vi "Time Delay.vi"(0 "Waiting Time(S)":u32, 1 "Pop Messige":string="Time Remaining:", 3 "error in (no error)":errorcluster) -> (10 "error out":errorcluster)   [LabVIEW 2020]
panel:
  out "String":string
  out "Horizontal Progress Bar":u32(slide) min=30 max=30000 scale=-1.0..10.0
  in  "Stop":bool
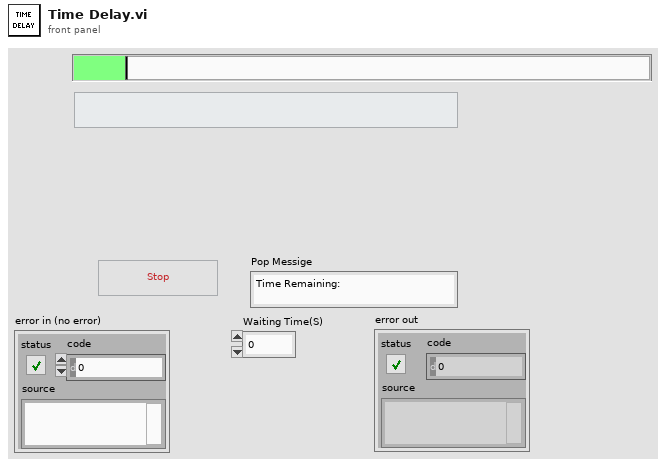
[diagram p1: front panel]
types:
  T1 = typedef "imagedata.ctl" = cluster{"image type":i32, "image depth":i32, "image":u8[], "mask":u8[], "colors":u32[], "Rectangle":cluster{"left":i16, "top":i16, "right":i16, "bottom":i16}}
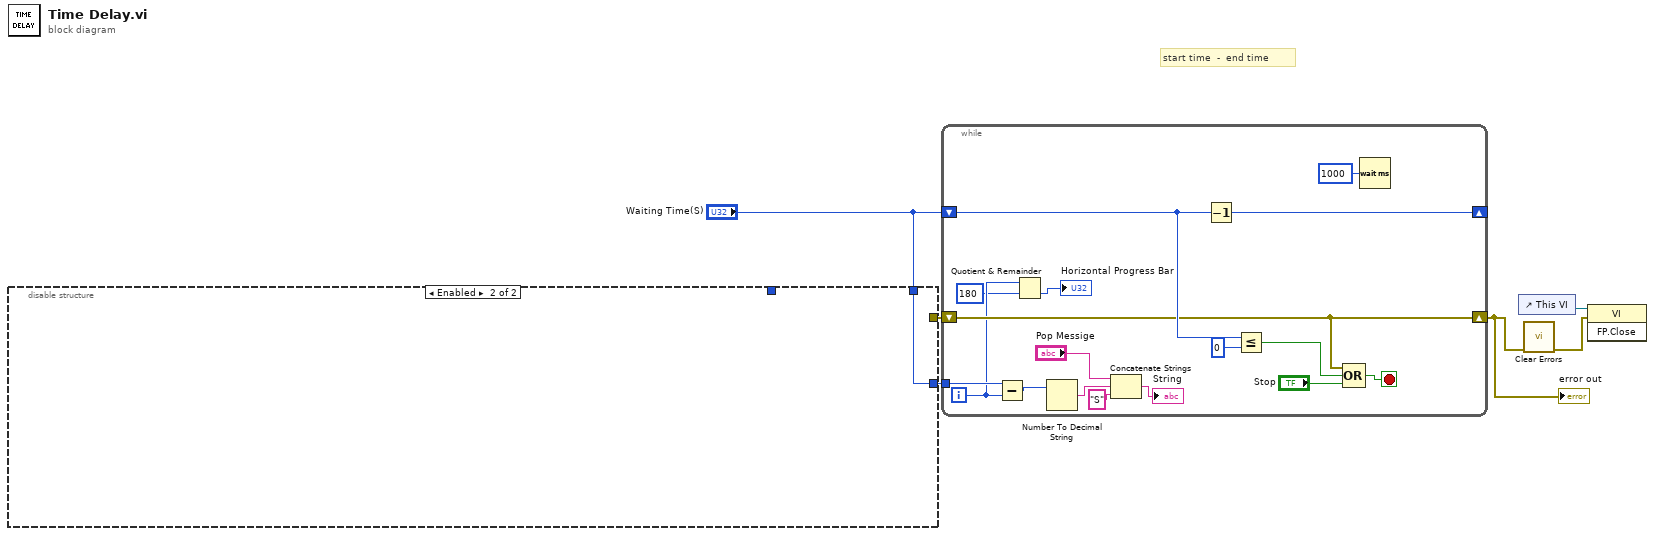
[diagram p0: block diagram]
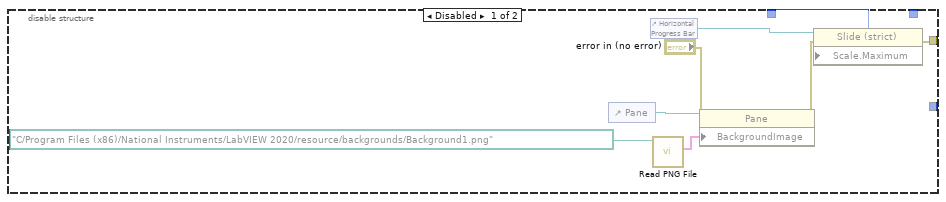
[diagram p2: hidden frame]
diagram:
  # "start time  -  end time"
  n1 = disable-structure shown="Enabled" {
    disable-tunnel: [w14 _] -> w6
    disable-tunnel: _ -> [w12 _]
    disable-tunnel: [_ w15] -> w2
    disable-tunnel: "Waiting Time(S)" -> [_ w15]
    frame Disabled {
      n2 = control-ref of="Pane"() -> (w11:refnum<vi>)
      n3 = control-ref of="Horizontal Progress Bar"() -> (w13:refnum<vi>)
      n4 = call <vilib>:"Read PNG File.vi"("path to PNG file"=path "C:/Program Files (x86)/National Instruments/LabVIEW 2020/resource/backgrounds/Background1.png") -> ("image data"=w10:T1)  [unwired: 8 in, 2 out]
      n5 = property class="Pane"(reference=w11, error in="error in (no error)", "BackgroundImage"=w10) -> (error out=w7:errorcluster)  [unwired: 1 out]
      n6 = property class="Slide (strict)"(reference=w13, error in=w7, "Scale.Maximum"=w12) -> (error out=w14:errorcluster)  [unwired: 1 out]
    }
    frame Enabled {
    }
  }
  n7 = while {
    shift-right: [w27] -> _
    shift-left: "Waiting Time(S)" -> [w22]
    shift-right: [w19] -> w4
    shift-left: w6 -> [w19]
    tunnel: w2 -> [w20]
    i -> [w18]
    stop <- w28 stop-if-true
    n8 = Subtract(x=w20, y=w18) -> (x-y=w21:u32)
    n9 = Quotient & Remainder(x=w18, y=180) -> (floor(x/y)=→"Horizontal Progress Bar":i32)  [unwired: 1 out]
    n10 = Number To Decimal String(number=w21) -> (decimal integer string=w26:string)  [unwired: 1 in]
    n11 = Concatenate Strings("Pop Messige", w26, "S" ("string")) -> (→"String":string)
    n12 = Decrement(x=w22) -> (x-1=w27:u32)
    n13 = Less Or Equal?(x=w22, y=u32 0) -> (x <= y?=w30:bool)
    n14 = Compound Arithmetic op=OR(w19, w30, "Stop") -> (w28:bool)
    n15 = Wait (ms)(milliseconds to wait=u32 1000) -> ()  [unwired: 1 out]
  }
  "error out" <- w4
  n16 = control-ref of="This VI"() -> (w5:refnum<vi>)
  n17 = call <vilib>:"Clear Errors.vi"("error in (no error)"=w4) -> ("error out"=w3:errorcluster)  [unwired: 5 in, 1 out]
  n18 = invoke class="VI" method="FP.Close"(reference=w5, error in=w3) -> ()  [unwired: 1 in, 3 out]
